vi "Leaf.vi"() -> ()   [LabVIEW 2018]
uses:
  Global_Telescopio.vi
panel:
  out "sendCommandShutter":bool
  out "ledFechando":bool
  in  "Lock Button":bool
  in  "ok":bool
  in  "Senha:":string
  out "String":string="\n\nNÍVEL CRÍTICO DE UMIDADE\n\n\nPOR FAVOR FECHE A TRAPEIRA \n\nEntre em contato com o assistente noturno."
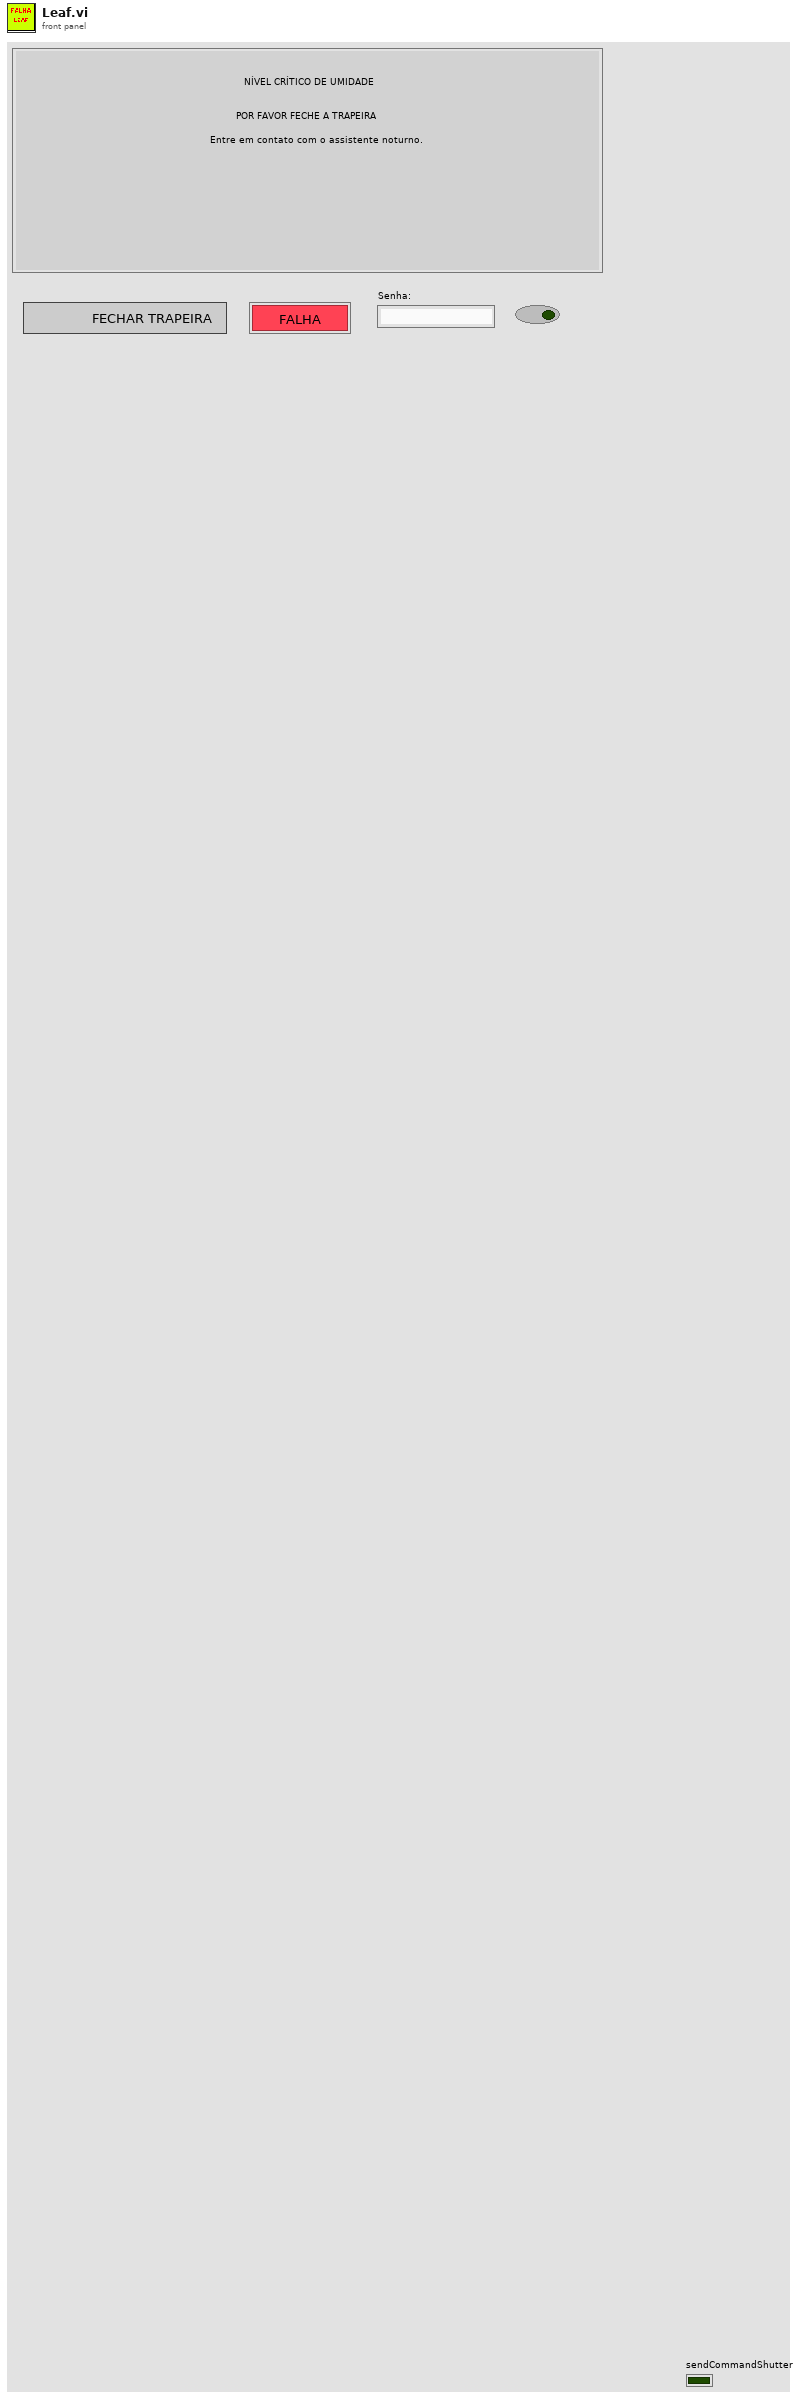
[diagram p1: front panel]
types:
  T1 = enum8{"Enabled", "Disabled", "Disabled and Grayed Out"}
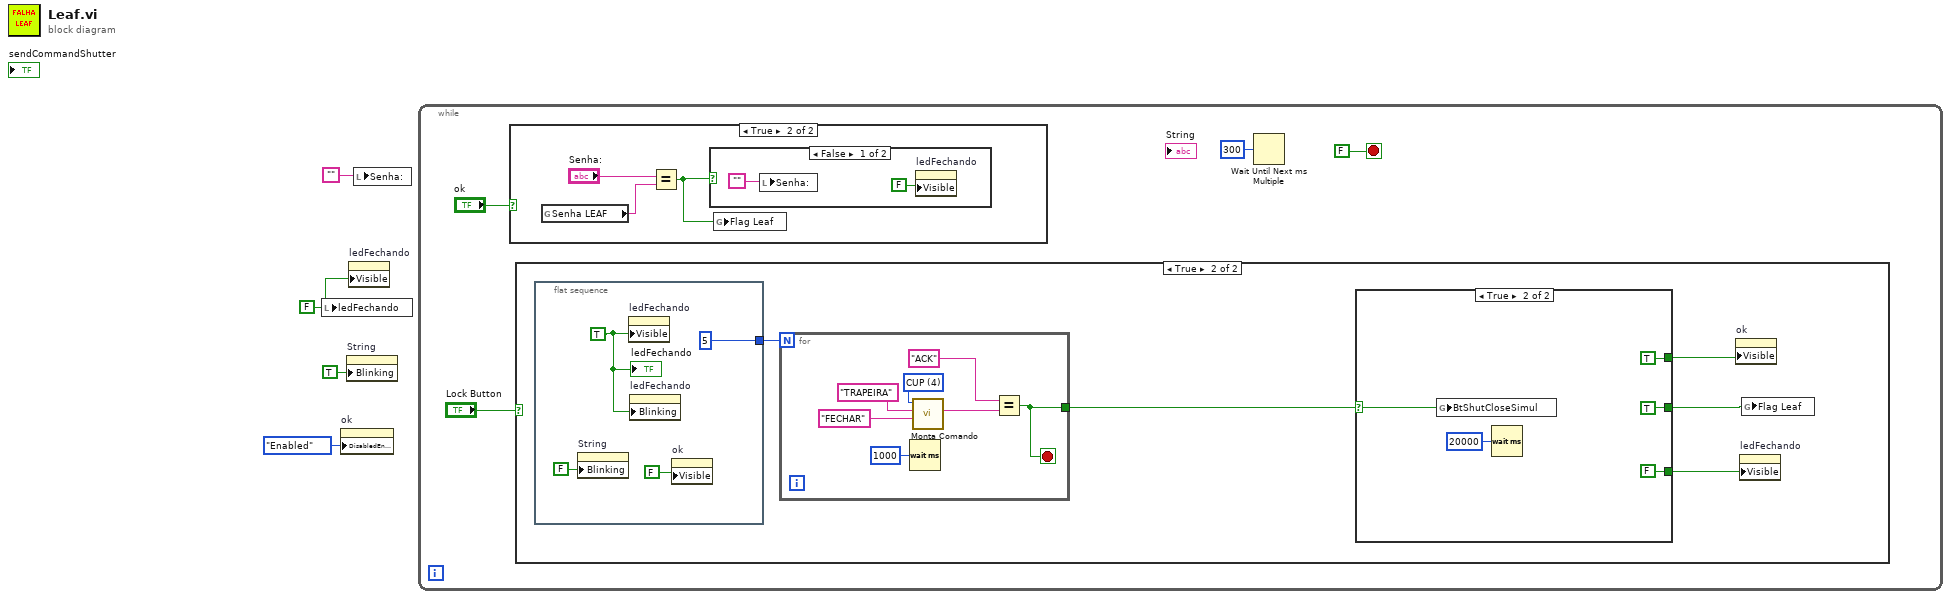
[diagram p0: block diagram]
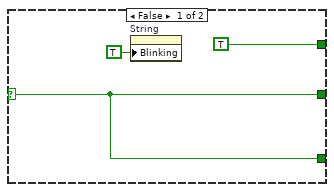
[diagram p3: hidden frame]
diagram:
  w3 = FALSE
  n1 = local write "ledFechando"(w3) -> ()
  n2 = property on="ok" class="Bool"("DisabledEnum"=T1."Enabled" ("Disabled")) -> ()  [unwired: 2 in, 2 out]
  n3 = property on="String" class="Str"("Blinking"=TRUE) -> ()  [unwired: 2 in, 2 out]
  n4 = property on="ledFechando" class="Bool (strict)"("Visible"=w3) -> ()  [unwired: 2 in, 2 out]
  n5 = local write "Senha:"("") -> ()
  n6 = while {
    stop <- FALSE stop-if-true
    n7 = case shown="True" "ok" {
      frame False {
      }
      frame True {
        n8 = global read "Global_Telescopio.vi" "Senha LEAF"() -> (w34:string)
        n9 = Equal?(x="Senha:", y=w34) -> (x = y?=w33:bool)
        n10 = case shown="False" w33 {
          frame False {
            n11 = local write "Senha:"("") -> ()
            n12 = property on="ledFechando" class="Bool (strict)"("Visible"=FALSE) -> ()  [unwired: 2 in, 2 out]
          }
          frame True {
          }
        }
        n13 = global write "Global_Telescopio.vi" "Flag Leaf"(w33) -> ()
      }
    }
    n14 = case shown="True" "Lock Button" {
      frame False {
      }
      frame True {
        n15 = flat-sequence {
          tunnel: [5] -> w13
          frame #0 {
            w17 = TRUE
            n16 = property on="String" class="Str"("Blinking"=FALSE) -> ()  [unwired: 2 in, 2 out]
            n17 = property on="ledFechando" class="Bool (strict)"("Visible"=w17) -> ()  [unwired: 2 in, 2 out]
            n18 = property on="ledFechando" class="Bool (strict)"("Blinking"=w17) -> ()  [unwired: 2 in, 2 out]
            n19 = property on="ok" class="Bool"("Visible"=FALSE) -> ()  [unwired: 2 in, 2 out]
            "ledFechando" <- w17
          }
        }
        n20 = for {
          N: w13 -> [_]
          tunnel: [w26] -> w9
          stop <- w26 stop-if-true
          w32 = u16 4 items=["ZERO", "AH", "DEC", "TUBO", "CUP"] ("Controlador")
          n21 = Wait (ms)(milliseconds to wait=u32 1000) -> ()  [unwired: 1 out]
          n22 = call "Monta Comando.vi"("Comando"="FECHAR", "Dispositivo"="TRAPEIRA" ("Comando"), "Controlador"=w32) -> ("Resposta"=w27:string)  [unwired: 2 in, 4 out]
          n23 = Equal?(x="ACK" ("Comando"), y=w27) -> (x = y?=w26:bool)
        }
        n24 = case shown="True" w9 {
          selector: w9 -> [w19 w21]
          tunnel: [w19 TRUE] -> w12
          tunnel: [TRUE TRUE] -> w11
          tunnel: [w19 FALSE] -> w10
          frame False {
            n25 = property on="String" class="Str"("Blinking"=TRUE) -> ()  [unwired: 2 in, 2 out]
          }
          frame True {
            n26 = global write "Global_Telescopio.vi" "BtShutCloseSimul"(w21) -> ()
            n27 = Wait (ms)(milliseconds to wait=u32 20000) -> ()  [unwired: 1 out]
          }
        }
        n28 = property on="ok" class="Bool"("Visible"=w11) -> ()  [unwired: 2 in, 2 out]
        n29 = property on="ledFechando" class="Bool (strict)"("Visible"=w10) -> ()  [unwired: 2 in, 2 out]
        n30 = global write "Global_Telescopio.vi" "Flag Leaf"(w12) -> ()
      }
    }
    n31 = Wait Until Next ms Multiple(millisecond multiple=u32 300) -> ()  [unwired: 1 out]
  }
